vi "Camera Tester - Calibration.vi"() -> ()   [LabVIEW 2020]
uses:
  <vilib>/vision/driver/IMAQdx.llb/IMAQdx Buffer Number Mode.ctl
  <vilib>/vision/driver/NI_Vision_Acquisition_Software.lvlib
panel:
  out "mm/pixel":dbl
  in  "Millimeters":dbl format="%#_13g"
  in  "Camera Name":refnum<k21> caption="IMAQdx Session"
  out "Image":T1(plugin-control)
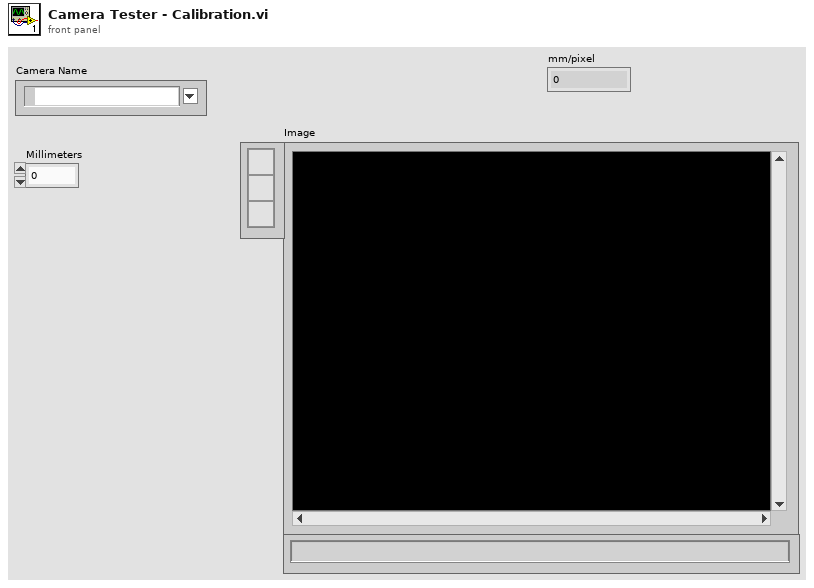
[diagram p1: front panel]
types:
  T1 = typedef "IMAQ Image.ctl" = refnum<image>
  T2 = typedef "IMAQdx.ctl" = refnum<k21>
  T3 = typedef "NI_Vision_Acquisition_Software.lvlib/IMAQdx Buffer Number Mode.ctl" = enum32{"Next", "Last", "Buffer Number", "Every", "Last New"}
  T4 = cluster{"Global Rectangle":i32[], "Contours":cluster{"Contour Type":u32, "ROI Type":u32, "Points":i32[]}[]}
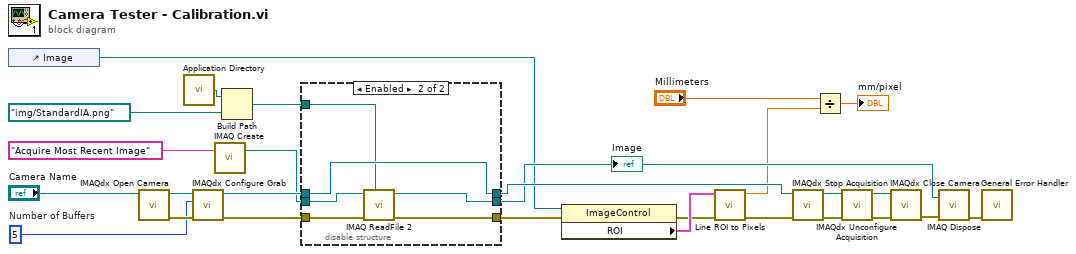
[diagram p0: block diagram]
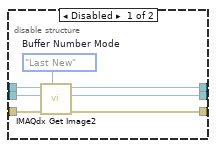
[diagram p2: hidden frame]
diagram:
  w17 = u32 5  # Number of Buffers
  n1 = control-ref of="Image"() -> (w4:refnum<vi>)
  n2 = call <vilib>:"IMAQdx Open Camera.vi"("Session In"="Camera Name") -> ("error out"=w19:errorcluster, "Session Out"=w20:T2)  [unwired: 2 in, 7 out]
  n3 = call <vilib>:"Application Directory.vi"() -> ("Application Directory"=w10:path)
  n4 = call <vilib>:"IMAQdx Configure Grab.vi"("error in"=w19, "Number of Buffers"=w17, "Session In"=w20) -> ("error out"=w15:errorcluster, "Session Out"=w16:T2)  [unwired: 7 in]
  n5 = call "IMAQ Create"("Image Name"="Acquire Most Recent Image") -> ("New Image"=w14:T1)  [unwired: 3 in, 2 out]
  n6 = Build Path(base path=w10, name or relative path=path "img/StandardIA.png") -> (appended path=w11:path)
  n7 = disable-structure shown="Enabled" {
    disable-tunnel: w16 -> [w33 w40]
    disable-tunnel: w15 -> [w32 w39]
    disable-tunnel: w14 -> [w31 w35]
    disable-tunnel: [w30 w40] -> w13
    disable-tunnel: [w29 w38] -> w2
    disable-tunnel: [w28 w37] -> w12
    disable-tunnel: w11 -> [_ w36]
    frame Disabled {
      w34 = IMAQdx_Buffer_Number_Mode."Last New"  # Buffer Number Mode
      n8 = call <vilib>:"IMAQdx Get Image2.vi"("Buffer Number Mode (Next)"=w34, "error in"=w32, "Image In"=w31, "Session In"=w33) -> ("error out"=w29:errorcluster, "Image Out"=w28:T1, "Session Out"=w30:T2)  [unwired: 4 in, 1 out]
    }
    frame Enabled {
      n9 = call "IMAQ ReadFile 2"("File Path"=w36, "error in (no error)"=w39, "Image"=w35) -> ("error out"=w38:errorcluster, "Image Out"=w37:T1)  [unwired: 4 in, 3 out]
    }
  }
  "Image" <- w12
  n10 = property class="ImageControl"(reference=w4, error in=w2) -> (error out=w1:errorcluster, "ROI"=w3:T4)  [unwired: 1 out]
  n11 = call "Line ROI to Pixels.vi"("error in (no error)"=w1, "ROI"=w3) -> ("error out"=w6:errorcluster, "pixel dist"=w5:dbl)  [unwired: 8 in]
  n12 = call <vilib>:"IMAQdx Stop Acquisition.vi"("error in"=w6, "Session In"=w13) -> ("error out"=w24:errorcluster, "Session Out"=w25:T2)  [unwired: 8 out]
  n13 = Divide(x="Millimeters", y=w5) -> (x/y=→"mm/pixel":dbl)
  n14 = call <vilib>:"IMAQdx Unconfigure Acquisition.vi"("error in"=w24, "Session In"=w25) -> ("error out"=w27:errorcluster, "Session Out"=w26:T2)  [unwired: 8 out]
  n15 = call <vilib>:"IMAQdx Close Camera.vi"("error in"=w27, "Session In"=w26) -> ("error out"=w23:errorcluster)  [unwired: 9 out]
  n16 = call "IMAQ Dispose"("Image"=w12, "error in (no error)"=w23) -> ("error out"=w22:errorcluster)  [unwired: 4 in]
  n17 = call <vilib>:"General Error Handler.vi"("error in (no error)"=w22) -> ()  [unwired: 2 in, 13 out]
